vi "Set Gear Ratio.vi"(8 "error in (no error)":errorcluster, 10 "Gear Ratio":dbl, 11 "Link In":refnum<class "NI_Robotics_Link.lvclass">) -> (0 "error out":errorcluster, 3 "Link Out":refnum<class "NI_Robotics_Link.lvclass">)   [LabVIEW 2017, in "NI_Robotics_Link.lvclass"]
uses:
  <vilib>/robotics/Kinematics/Link/NI_Robotics_Link.lvclass
  <vilib>/robotics/Kinematics/Link/NI_Robotics_Link.lvclass/NI_Robotics_Link.ctl
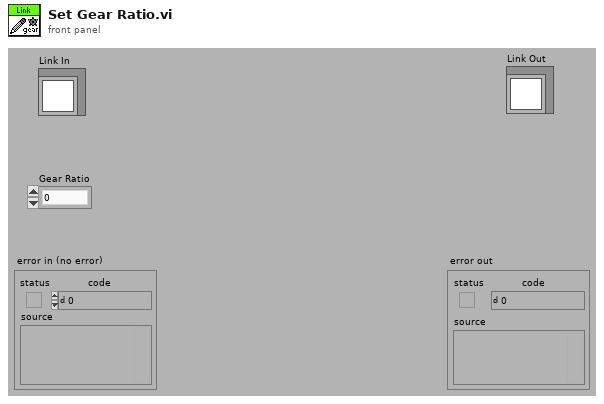
[diagram p1: front panel]
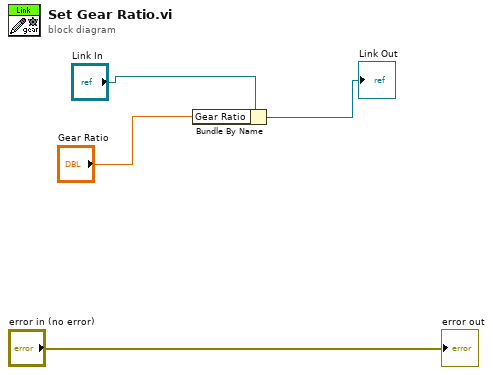
[diagram p0: block diagram]
diagram:
  n1 = Bundle By Name(cluster="Link In", "Gear Ratio"="Gear Ratio") -> (→"Link Out":refnum<class "NI_Robotics_Link.lvclass">)
  "error out" <- "error in (no error)"
